vi "GetClassNameAndVersion.vi"(8 "error in (no error)":errorcluster, 11 "Class":T3) -> (0 "error out":errorcluster, 3 "Class NameVer":T1)   [LabVIEW 2020, in "BlueSerialization.lvlib" / "BlueSerializer.lvclass"]
uses:
  BlueSerializer.lvclass
  ClassNameObj.ctl
  ClassNameAndVersion.ctl
  <vilib>/Utility/EditLVLibs/LibVersion.ctl
  <vilib>/Utility/EditLVLibs/LVClass/Get Mutation History.vi
  <vilib>/Utility/EditLVLibs/Edit LVLibs.lvlib
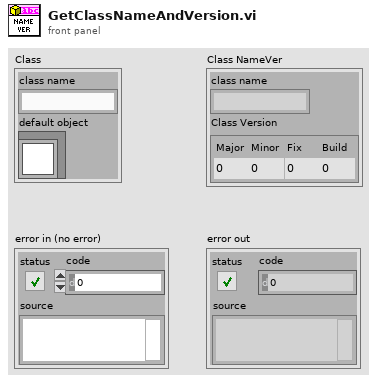
[diagram p1: front panel]
types:
  T1 = typedef "BlueSerialization.lvlib/BlueSerializer.lvclass/ClassNameAndVersion.ctl" = cluster{"class name":string, "Class Version":T2}
  T2 = typedef "Edit LVLibs.lvlib/LibVersion.ctl" = cluster{"Major":u16, "Minor":u16, "Fix":u16, "Build":u16}
  T3 = typedef "BlueSerialization.lvlib/BlueSerializer.lvclass/ClassNameObj.ctl" = cluster{"class name":string, "default object":refnum<class>}
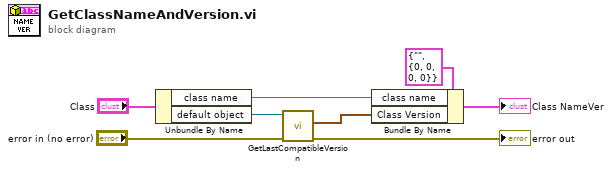
[diagram p0: block diagram]
diagram:
  n1 = Unbundle By Name("Class") -> ("class name"=w6:string, "default object"=w4:refnum<class>)
  n2 = call "GetLastCompatibleVersion.vi"("error in (no error)"="error in (no error)", "LabVIEW Object"=w4) -> ("error out"=→"error out":errorcluster, "Last Compatible Class Version"=w3:T2)  [unwired: 7 in, 1 out]
  n3 = Bundle By Name(cluster=T1 {"class name"="", "Class Version"={"Major"=0, "Minor"=0, "Fix"=0, "Build"=0}} ("Cluster"), "class name"=w6, "Class Version"=w3) -> (→"Class NameVer":T1)
